vi "Set Random Tracks.vi"(10 "areas":i32, 11 "numTracks":i32) -> (2 "areas out":i32, 3 "function return":u32)   [LabVIEW 2018, in "Copy of Andor SDK.lvlib"]
doc: "EXPNETTYPE unsigned int WINAPI SetRandomTracks(int numTracks, int * areas);"
uses:
  Copy of Andor SDK.lvlib
  <userlib>/Andor SDK/ATMCD32D.dll
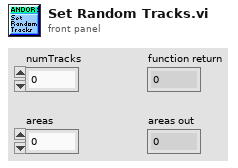
[diagram p1: front panel]
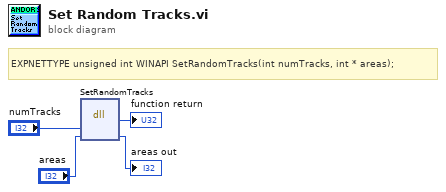
[diagram p0: block diagram]
diagram:
  # "EXPNETTYPE unsigned int WINAPI SetRandomTracks(int numTracks, int * areas);"
  n1 = dll-call lib="C:/Program Files (x86)/National Instruments/LabVIEW 2018/user.lib/Andor SDK/ATMCD32D.*" fn="SetRandomTracks"("numTracks"="numTracks", "areas"="areas") -> (→"function return":u32, "areas"=→"areas out":i32)  [unwired: 4 in, 2 out]
